vi "VFD-mode-select.vi"(8 "Est/TAS IN":bool, 10 "Warning\nSent? IN":bool, 11 "VFD \nMode\nSelect":bool=TRUE) -> (0 "EST/TAS out":bool, 1 "Warning\nSent? OUT":bool, 2 "PID Mode Indc":bool, 3 "FRQ Indc":bool)   [LabVIEW 2025]
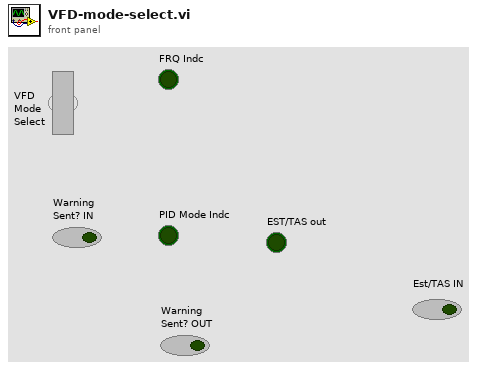
[diagram p1: front panel]
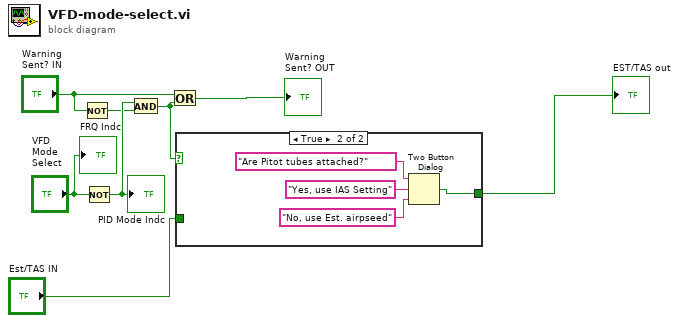
[diagram p0: block diagram]
diagram:
  n1 = Not(x="Warning\nSent? IN") -> (.not. x?=w4:bool)
  n2 = Not(x="VFD \nMode\nSelect") -> (.not. x?=w5:bool)
  "PID Mode Indc" <- w5
  n3 = And(x=w5, y=w4) -> (x .and. y?=w6:bool)
  n4 = Or(x="Warning\nSent? IN", y=w6) -> (x .or. y?=→"Warning\nSent? OUT":bool)
  n5 = case shown="True" w6 {
    tunnel: [w9 w10] -> w2
    tunnel: "Est/TAS IN" -> [w9 _]
    frame False {
    }
    frame True {
      n6 = Two Button Dialog(message="Are Pitot tubes attached?", 1:"No, use Est. airpseed" ("F button name (\"Cancel\")"), 2:"Yes, use IAS Setting" ("T button name (\"OK\")")) -> (T button?=w10:bool)
    }
  }
  "EST/TAS out" <- w2
  "FRQ Indc" <- "VFD \nMode\nSelect"
